vi "Read CSM API By CSM-VI.vi"(6 "Config Path":path, 8 "Error In":errorcluster caption="Error in (no error)", 11 "CSM VI":string) -> (0 "Error Out":errorcluster, 3 "Array":string[](array[string]))   [LabVIEW 2017, in "CSM-Helper API with lvcsm Support.lvlib"]
uses:
  CSM-Helper API with lvcsm Support.lvlib
  lvcsmFile/lvcsm File Support.lvlib
  CSM-Helper.lvclass
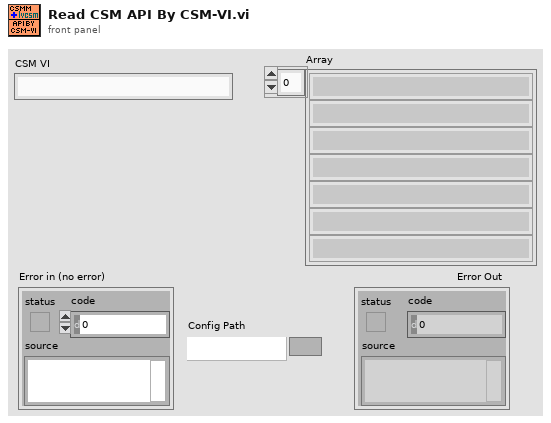
[diagram p1: front panel]
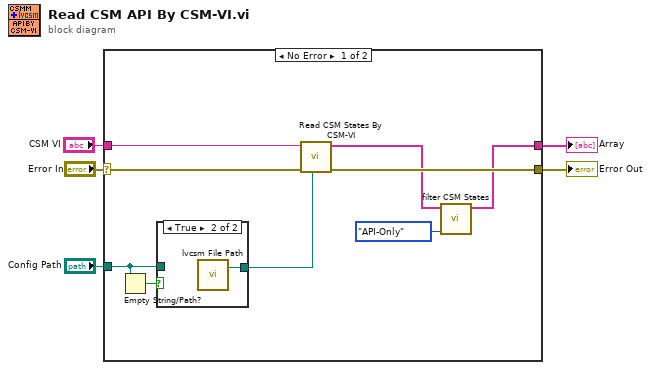
[diagram p0: block diagram]
diagram:
  n1 = case shown="No Error" "Error In" {
    selector: "Error In" -> [w11 w17]
    tunnel: [w10 w17] -> w4
    tunnel: "Config Path" -> [w14 _]
    tunnel: [w7 _] -> w2
    tunnel: "CSM VI" -> [w12 _]
    frame No Error {
      n2 = Empty String/Path?(string/path=w14) -> (empty?=w13:bool)
      n3 = case shown="True" w13 {
        tunnel: [w15 w16] -> w9
        tunnel: w14 -> [w15 _]
        frame False {
        }
        frame True {
          n4 = call "lvcsm File Path.vi"() -> ("Appended Path"=w16:path)  [unwired: 3 in]
        }
      }
      n5 = call "Read CSM States By CSM-VI.vi"("Config Path"=w9, "Error In"=w11, "CSM VI"=w12) -> ("Error Out"=w10:errorcluster, "Array"=w8:string[])  [unwired: 7 in]
      n6 = call "filter CSM States.vi"("Interface-Filter"=enum16{"API-Only", "UserDef States", "All"}."API-Only", "Array"=w8) -> ("filtered array"=w7:string[])  [unwired: 9 in]
    }
    frame Error {
    }
  }
  "Error Out" <- w4
  "Array" <- w2
